vi "Calculate State.vi"(8 "error in (no error)":errorcluster, 11 "Path":path) -> (0 "error out":errorcluster, 3 "digest":string)   [LabVIEW 2020, in "Test Finder.lvclass"]
uses:
  Test Finder.lvclass
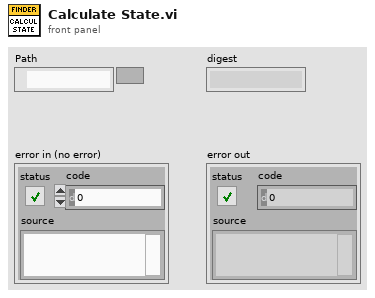
[diagram p1: front panel]
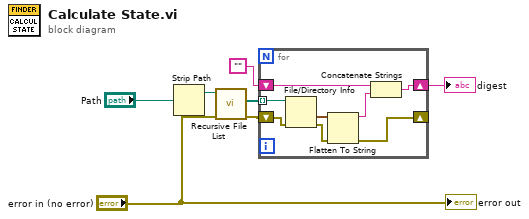
[diagram p0: block diagram]
diagram:
  n1 = Strip Path(path="Path") -> (stripped path=w4:path)  [unwired: 1 out]
  n2 = call <vilib>:"Recursive File List.vi"("error in (no error)"="error in (no error)", "Folder Path"=w4) -> ("error out"=w2:errorcluster, "All Files in Dir"=w6:path[])  [unwired: 5 in, 3 out]
  n3 = for {
    tunnel: w6 -> [w15] mode=indexing
    shift-right: [w12] -> w3
    shift-left: "" ("data string") -> [w11]
    shift-right: [w8] -> _
    shift-left: w2 -> [w10]
    n4 = File/Directory Info(path=w15, error in=w10) -> (last mod=w13:timestamp, error out=w9:errorcluster)  [unwired: 5 out]
    n5 = Flatten To String(anything=w13, error in (no error)=w9) -> (data string=w14:string, error out=w8:errorcluster)  [unwired: 2 in, 1 out]
    n6 = Concatenate Strings(w11, w14) -> (w12:string)
  }
  "digest" <- w3
  "error out" <- "error in (no error)"
